vi "gyro_hand_display.vi"() -> ()   [LabVIEW 2019]
uses:
  SubVIs/Gyro_Reader/Controls/gyro_control_measurement_settings.ctl
panel:
  in  "Tab Control":enum32{"File IO", "Selection", "Time", "SNR"}(tab)
  in  "Missing GPX file":bool
  in  "Missing Hand file":bool
  in  "Missing Ship file":bool
  in  "GPX path":path
  in  "Hand path":path
  in  "Ship path":path
  in  "Old Akti File":bool
  out "hand data":waveform(dbl)[](graph)
  out "ship data":waveform(dbl)[](graph)
  in  "Sec":dbl=60.0
  in  "Start Cursor":timestamp
  in  "Reset Cursors":bool
  in  "GPS Offset":dbl
  out "GPS Graph":cluster{timestamp[], "Y":dbl[]}[](graph)
  in  "Read in Button":bool
  in  "Stop Button":bool
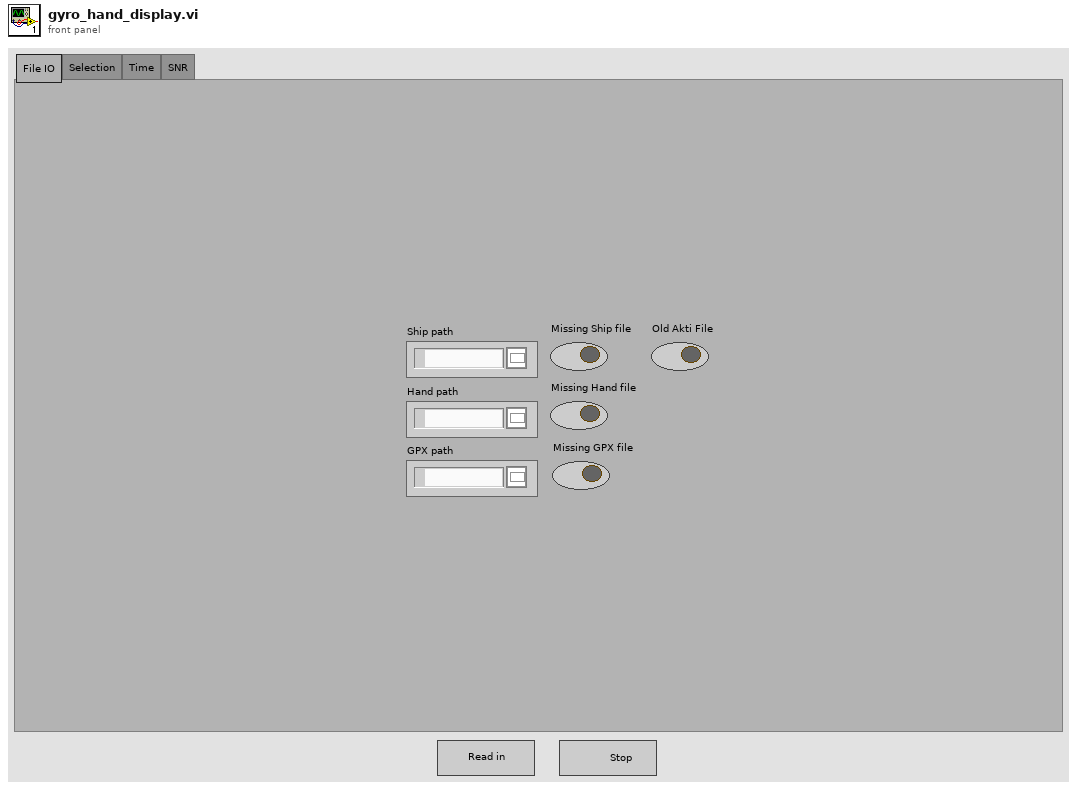
[diagram p1: front panel]
types:
  T1 = typedef "gyro_control_measurement_settings.ctl" = cluster{"# Pages":i32, "ODR":u8, "xlRange":u8, "gyroRange":u8, "id":u8, "Samplig Freq [Hz]":dbl, "xlRange in g":dbl, "gyroRange in dps":dbl}
  T2 = cluster{"IO Meta":cluster{"ship file missing?":bool, "hand file missing?":bool, "GPX file missing?":bool, "old akti file?":bool, "Start Time":timestamp, "GPS offset":dbl}, "Ship Data":cluster{"Ship Acceleration":waveform(dbl)[], "Ship Angular Velocity":waveform(dbl)[]}, "Hand Data":cluster{"Hand Acceleration":waveform(dbl)[], "Hand Angular Velocity":waveform(dbl)[]}, "Ship Meta":T1, "Hand Meta":T1, "GPS Data":cluster{"XY Speed data":cluster{"Array":timestamp[], "Array":dbl[]}, "Lat/Lon Position":cluster{"Array":timestamp[], "Array":dbl[], "Array":dbl[]}, "Position Graph":cluster{"X":dbl, "Y":dbl}[]}}
  T3 = typedef "LVRangeTypeDef.ctl" = cluster{"Minimum":dbl, "Maximum":dbl, "Increment":dbl, "Minor Increment":dbl, "Start":dbl}
  T4 = typedef "control_all_in_one_package.ctl" = cluster{"memory structure":T5, "actigraph settings":T6, "time informations":T7, "measurement data":T8}
  T5 = typedef "control_memory_structure.ctl" = cluster{"length of metadata [byte]":i32, "length of page [byte]":i32, "length of measurement data on page [byte]":i32, "length of dataset [byte]":i32}
  T6 = typedef "control_measurement_settings.ctl" = cluster{"sampling frequency [Hz]":dbl, "measurement interval [± g]":i32, "high precision?":bool, "number of pages":i32, "rate code":i32, "range code":i32, "id":i32}
  T7 = typedef "control_time_informations.ctl" = cluster{"starting time":timestamp, "ending time":timestamp, "dt[s]":dbl, "sampling rate [Hz]":dbl, "length":dbl}
  T8 = typedef "control_measurement_data.ctl" = cluster{"number of samples per axis":i32, "timestamp array":dbl[], "offset array":dbl[], "x, y, z axis data":waveform(dbl)[], "normalised magnitude of acceleartion vectors":waveform(dbl), "calibration coefficients":T9, "statistics":T10, "battery voltage":waveform(dbl), "magnitude of acceleartion vectors":waveform(dbl)}
  T9 = typedef "control_calibration_coefficients.ctl" = cluster{"Sx":dbl, "Ox":dbl, "Sy":dbl, "Oy":dbl, "Sz":dbl, "Oz":dbl}
  T10 = typedef "control_statistics.ctl" = cluster{"mean of x axis acceleration":dbl, "standard devation of x axis acceleration":dbl, "mean of y axis acceleration":dbl, "standard devation of y axis acceleration":dbl, "mean of z axis acceleration":dbl, "standard devation of z axis acceleration":dbl, "mean of normalised magnitude of acceleration":dbl, "standard devation of normalised magnitude of acceleration":dbl}
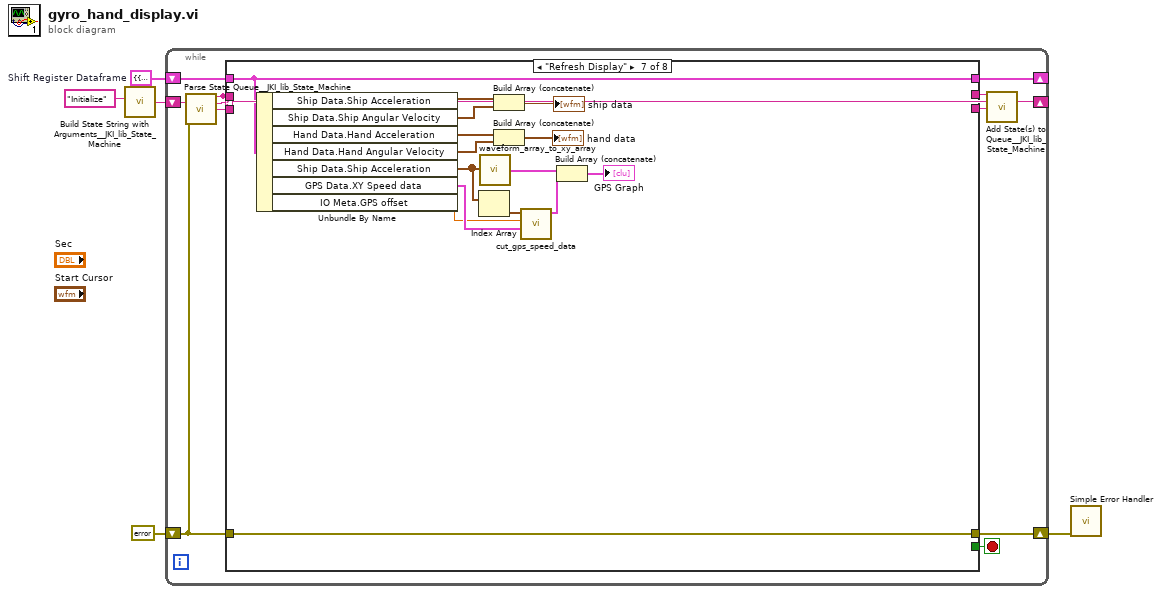
[diagram p0: block diagram]
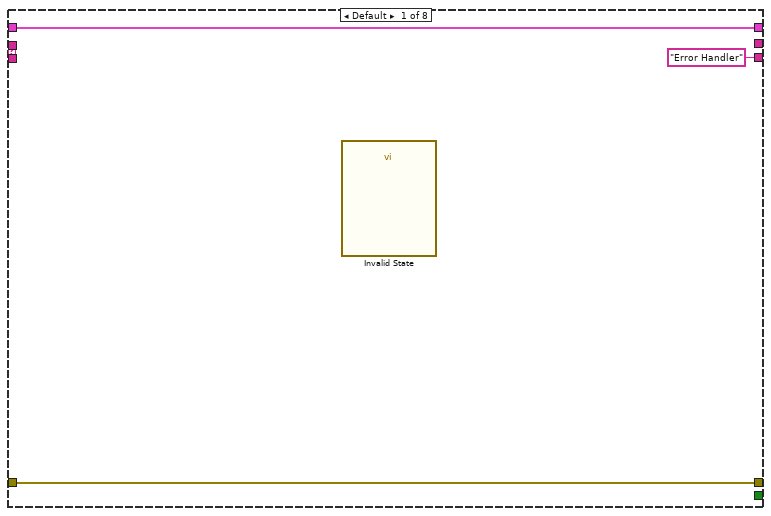
[diagram p2: hidden frame]
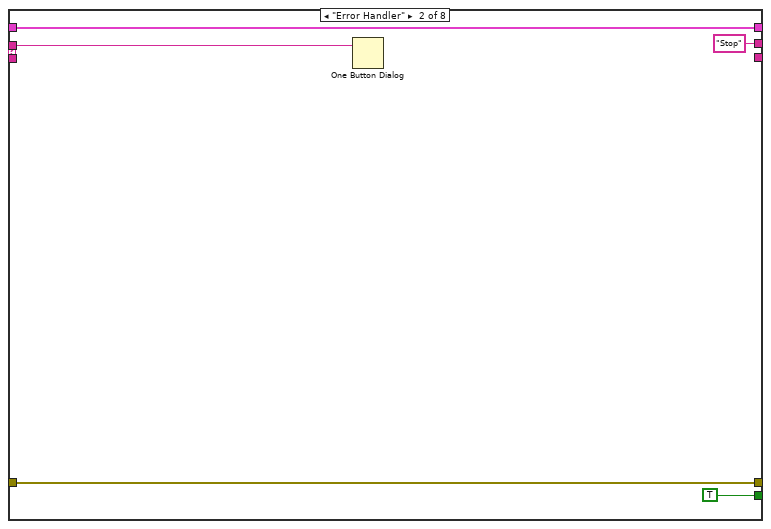
[diagram p3: hidden frame]
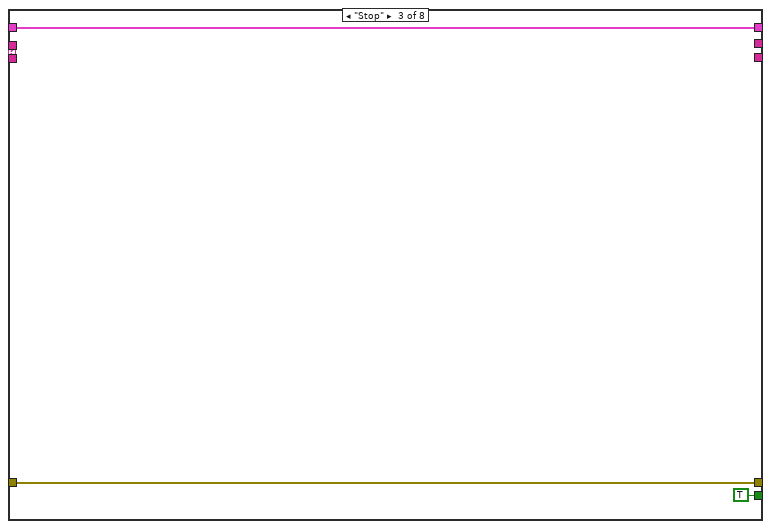
[diagram p4: hidden frame]
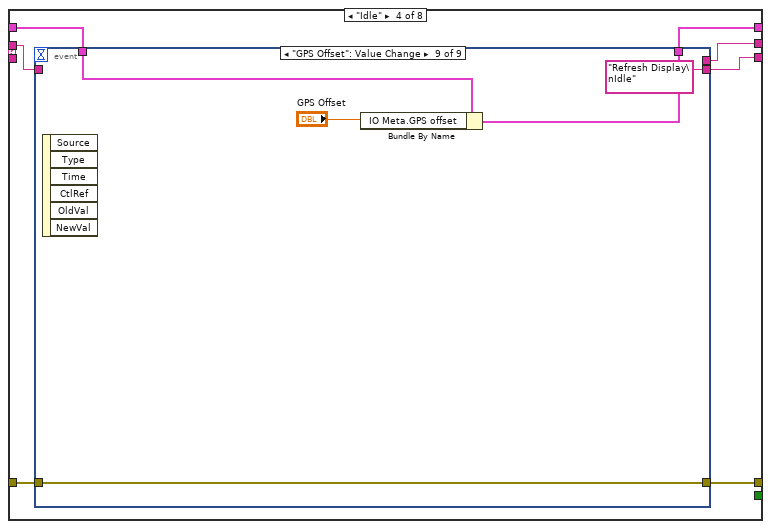
[diagram p5: hidden frame]
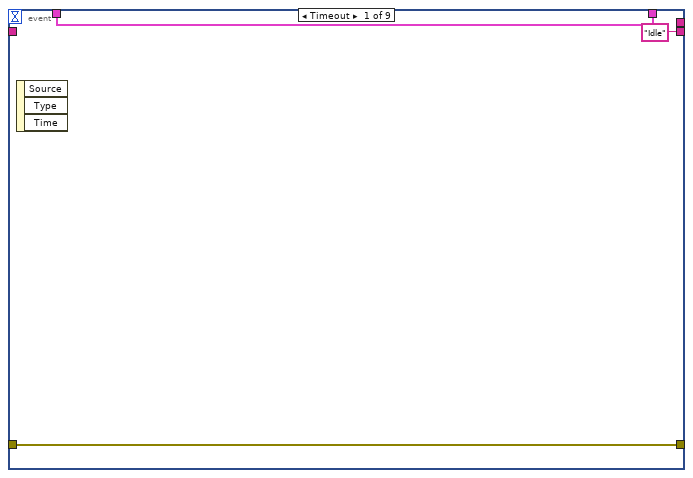
[diagram p6: hidden frame]
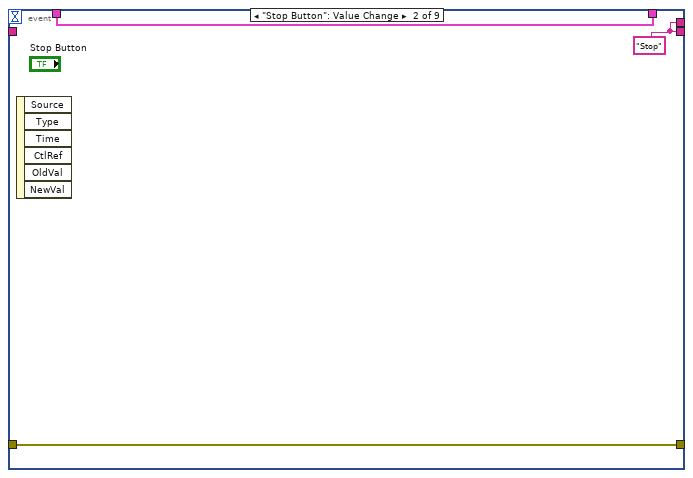
[diagram p7: hidden frame]
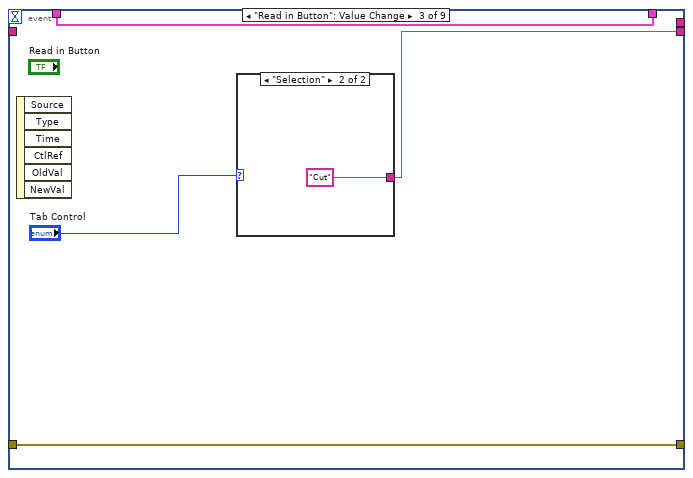
[diagram p8: hidden frame]
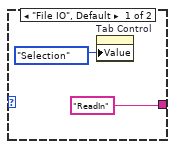
[diagram p9: hidden frame]
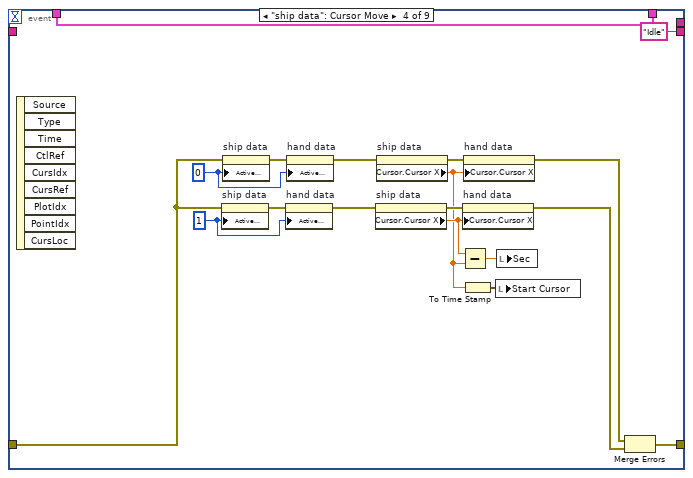
[diagram p10: hidden frame]
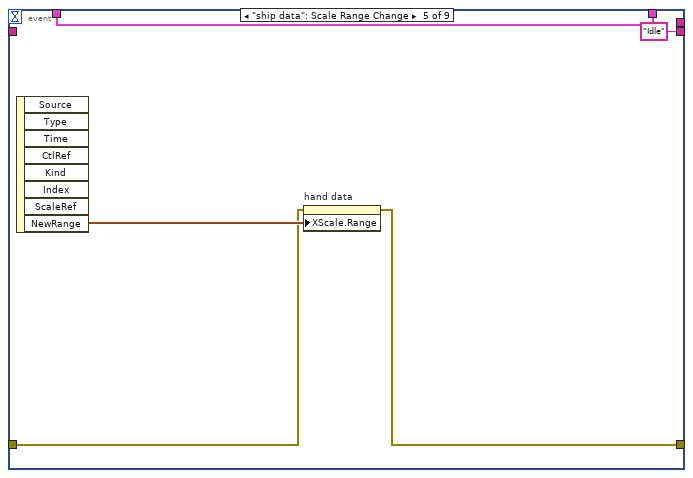
[diagram p11: hidden frame]
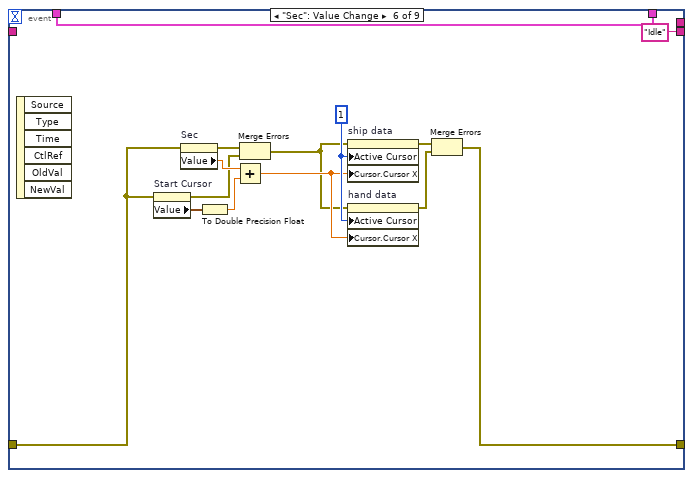
[diagram p12: hidden frame]
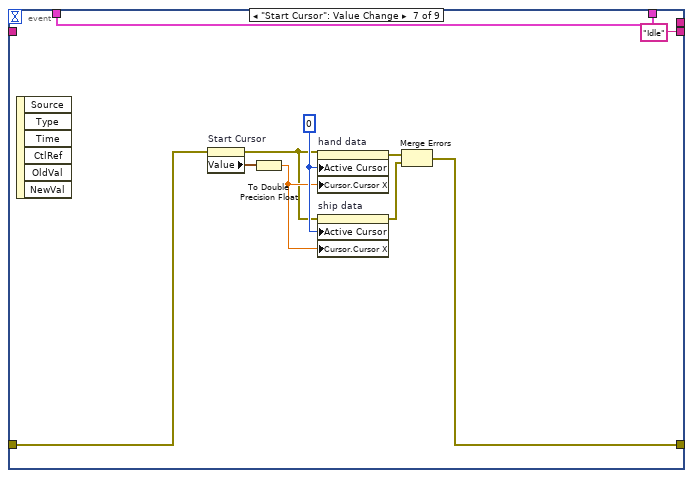
[diagram p13: hidden frame]
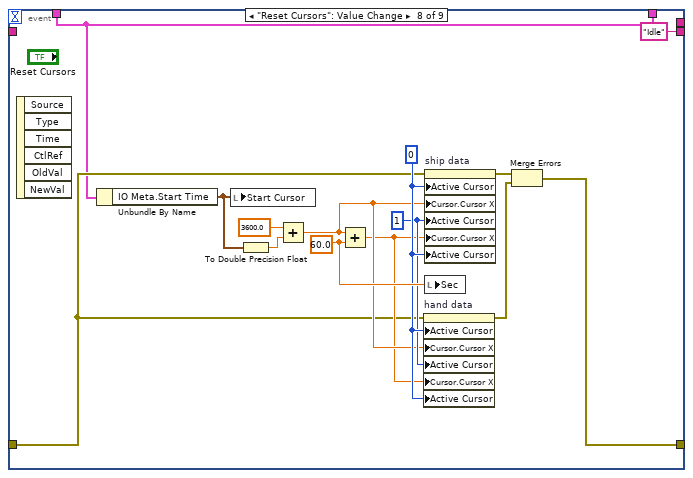
[diagram p14: hidden frame]
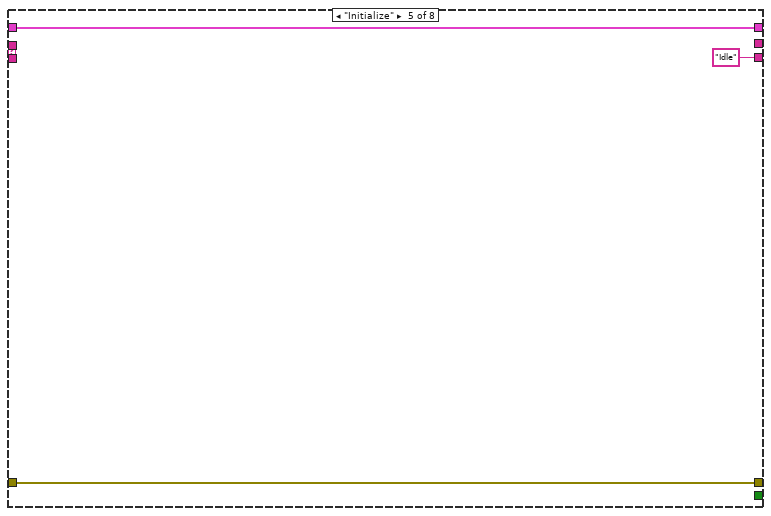
[diagram p15: hidden frame]
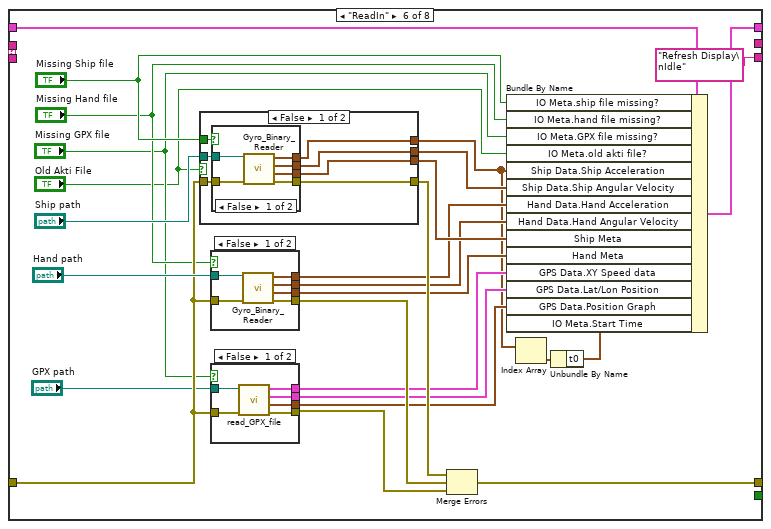
[diagram p16: hidden frame]
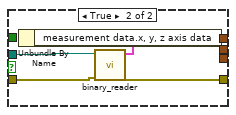
[diagram p20: hidden frame]
diagram:
  w1 = T2 {"IO Meta"={"ship file missing?"=TRUE, "hand file missing?"=TRUE, "GPX file missing?"=TRUE, "old akti file?"=FALSE, "Start Time"=timestamp(0 s since 1904-01-01), "GPS offset"=0.0}, "Ship Data"={"Ship Acceleration"=[], "Ship Angular Velocity"=[]}, "Hand Data"={"Hand Acceleration"=[], "Hand Angular Velocity"=[]}, "Ship Meta"={"# Pages"=0, "ODR"=0, "xlRange"=0, "gyroRange"=0, "id"=0, "Samplig Freq [Hz]"=9.980607627666451, "xlRange in g"=0.0, "gyroRange in dps"=0.0}, "Hand Meta"={"# Pages"=0, "ODR"=0, "xlRange"=0, "gyroRange"=0, "id"=0, "Samplig Freq [Hz]"=9.980607627666451, "xlRange in g"=0.0, "gyroRange in dps"=0.0}, "GPS Data"={"XY Speed data"={"Array"=[], "Array"=[]}, "Lat/Lon Position"={"Array"=[], "Array"=[], "Array"=[]}, "Position Graph"=[]}}  # Shift Register Dataframe
  n1 = call <vilib>:"Build State String with Arguments__JKI_lib_State_Machine.vi"("State"="Initialize") -> ("State with Arguments"=w5:string)  [unwired: 5 in]
  n2 = while {
    shift-right: [w14] -> w2
    shift-left: errorcluster {"status"=FALSE, "code"=0, "source"=""} ("error in (no error)") -> [w15]
    shift-right: [w7] -> _
    shift-left: w5 -> [w16]
    shift-right: [w9] -> _
    shift-left: w1 -> [w10]
    stop <- w17 stop-if-true
    n3 = call <vilib>:"Parse State Queue__JKI_lib_State_Machine.vi"("State Queue"=w16, "Error In (no error)"=w15) -> ("Remaining States"=w12:string, "Current State"=w13:string, "Arguments"=w11:string)  [unwired: 11 in]
    n4 = case shown="\"Refresh Display\"" w13 {
      tunnel: [_ TRUE TRUE _ _ _ _ _] -> w17
      tunnel: [w20 w24 w28 w35 w116 w141 w190 w192] -> w14
      tunnel: w15 -> [w20 w24 w28 w34 w116 w138 w190 w192]
      tunnel: w12 -> [_ w21 _ w33 _ _ _ _]
      tunnel: w11 -> [_ _ _ _ _ _ _ _]
      tunnel: w10 -> [w19 w23 w26 w30 w115 w117 w189 w193]
      tunnel: [w19 w23 w26 w29 w115 w134 w189 w193] -> w9
      tunnel: ["Error Handler" ("States Out") _ _ w32 "Idle" ("State(s) at Back (\"\")") "Refresh Display\nIdle" ("State(s) at Back (\"\")") _ "Idle" ("States Out")] -> w8
      tunnel: [_ "Stop" ("States Out") _ w31 _ _ _ _] -> w6
      frame Default {
        n5 = call "Invalid State"() -> ()  [unwired: 10 in, 2 out]
      }
      frame "Error Handler" {
        n6 = One Button Dialog(message=w21) -> ()  [unwired: 1 in, 1 out]
      }
      frame "Stop" {
      }
      frame "Idle" {
        n7 = event shown="[8] \"GPS Offset\": Value Change" {
          selector: _ -> [_ _ _ _ _ _ _ _ _]
          dyn-events: _ -> [_ _ _ _ _ _ _ _ _]
          timeout: _ -> [_ _ _ _ _ _ _ _ _]
          tunnel: w33 -> [_ _ _ _ _ _ _ _ _]
          tunnel: ["Idle" ("Remaining States") w40 w43 "Idle" ("Remaining States") "Idle" ("Remaining States") "Idle" ("Remaining States") "Idle" ("Remaining States") "Idle" ("Remaining States") "Refresh Display\nIdle" ("Remaining States")] -> w32
          tunnel: [w38 w41 w45 w58 w67 w78 w90 w96 w109] -> w35
          tunnel: w34 -> [w38 w41 w45 w60 w68 w72 w87 w99 w109]
          tunnel: [_ w40 _ _ _ _ _ _ _] -> w31
          tunnel: w30 -> [w36 w39 w42 w49 w66 w71 w85 w95 w113]
          tunnel: [w36 w39 w42 w49 w66 w71 w85 w95 w111] -> w29
          event Timeout {
            n8 = event-data() -> ()  [unwired: 1 in, 3 out]
          }
          event "Stop Button": Value Change {
            w40 = "Stop" ("Remaining States")
            n9 = event-data() -> ()  [unwired: 1 in, 6 out]
          }
          event "Read in Button": Value Change {
            n10 = event-data() -> ()  [unwired: 1 in, 6 out]
            n11 = case shown="\"Selection\"" "Tab Control" {
              tunnel: ["ReadIn" ("Remaining States") "Cut" ("Remaining States")] -> w43
              frame "File IO", Default {
                n12 = property on="Tab Control" class="TabCtl (strict)"("Value"=enum32{"File IO", "Selection", "Time", "SNR"}."Selection" ("Tab Control")) -> ()  [unwired: 2 in, 2 out]
              }
              frame "Selection" {
              }
            }
          }
          event "ship data": Cursor Move {
            w55 = 1
            w54 = 0
            n13 = event-data() -> ()  [unwired: 1 in, 9 out]
            n14 = property on="ship data" class="WFGraph (strict)"(error in=w60, "Active Cursor"=w55) -> (error out=w59:errorcluster)  [unwired: 1 in, 1 out]
            n15 = property on="ship data" class="WFGraph (strict)"("Active Cursor"=w54) -> ()  [unwired: 2 in, 2 out]
            n16 = property on="hand data" class="WFGraph (strict)"(error in=w59, "Active Cursor"=w55) -> (error out=w62:errorcluster)  [unwired: 1 in, 1 out]
            n17 = property on="hand data" class="WFGraph (strict)"(error in=w60, "Active Cursor"=w54) -> (error out=w64:errorcluster)  [unwired: 1 in, 1 out]
            n18 = property on="ship data" class="WFGraph (strict)"(error in=w62) -> (error out=w61:errorcluster, "Cursor.Cursor X"=w52:dbl)  [unwired: 1 in, 1 out]
            n19 = property on="ship data" class="WFGraph (strict)"(error in=w64) -> (error out=w65:errorcluster, "Cursor.Cursor X"=w50:dbl)  [unwired: 1 in, 1 out]
            n20 = Subtract(x=w52, y=w50) -> (x-y=w53:dbl)
            n21 = property on="hand data" class="WFGraph (strict)"(error in=w61, "Cursor.Cursor X"=w52) -> (error out=w56:errorcluster)  [unwired: 1 in, 1 out]
            n22 = To Time Stamp(1:w50) -> (0:w51:timestamp)
            n23 = property on="hand data" class="WFGraph (strict)"(error in=w65, "Cursor.Cursor X"=w50) -> (error out=w57:errorcluster)  [unwired: 1 in, 1 out]
            n24 = local write "Start Cursor"(w51) -> ()
            n25 = local write "Sec"(w53) -> ()
            n26 = Merge Errors(w57, w56) -> (w58:errorcluster)
          }
          event "ship data": Scale Range Change {
            n27 = event-data() -> ("NewRange"=w70:T3)  [unwired: 1 in, 7 out]
            n28 = property on="hand data" class="WFGraph (strict)"(error in=w68, "XScale.Range"=w70) -> (error out=w67:errorcluster)  [unwired: 1 in, 1 out]
          }
          event "Sec": Value Change {
            w82 = u32 1 ("Active Cursor")
            n29 = event-data() -> ()  [unwired: 1 in, 6 out]
            n30 = property on="Start Cursor" class="AbsTime (strict)"(error in=w72) -> (error out=w73:errorcluster, "Value"=w74:timestamp)  [unwired: 1 in, 1 out]
            n31 = property on="Sec" class="DigNum (strict)"(error in=w72) -> (error out=w77:errorcluster, "Value"=w83:dbl)  [unwired: 1 in, 1 out]
            n32 = To Double Precision Float(number=w74) -> (double precision float=w84:dbl)
            n33 = Add(x=w83, y=w84) -> (x+y=w81:dbl)
            n34 = Merge Errors(w77, w73) -> (w76:errorcluster)
            n35 = property on="ship data" class="WFGraph (strict)"(error in=w76, "Active Cursor"=w82, "Cursor.Cursor X"=w81) -> (error out=w80:errorcluster)  [unwired: 1 in, 1 out]
            n36 = property on="hand data" class="WFGraph (strict)"(error in=w76, "Active Cursor"=w82, "Cursor.Cursor X"=w81) -> (error out=w79:errorcluster)  [unwired: 1 in, 1 out]
            n37 = Merge Errors(w80, w79) -> (w78:errorcluster)
          }
          event "Start Cursor": Value Change {
            w92 = u32 0 ("Active Cursor")
            n38 = event-data() -> ()  [unwired: 1 in, 6 out]
            n39 = property on="Start Cursor" class="AbsTime (strict)"(error in=w87) -> (error out=w88:errorcluster, "Value"=w86:timestamp)  [unwired: 1 in, 1 out]
            n40 = To Double Precision Float(number=w86) -> (double precision float=w91:dbl)
            n41 = property on="hand data" class="WFGraph (strict)"(error in=w88, "Active Cursor"=w92, "Cursor.Cursor X"=w91) -> (error out=w93:errorcluster)  [unwired: 1 in, 1 out]
            n42 = property on="ship data" class="WFGraph (strict)"(error in=w88, "Active Cursor"=w92, "Cursor.Cursor X"=w91) -> (error out=w94:errorcluster)  [unwired: 1 in, 1 out]
            n43 = Merge Errors(w93, w94) -> (w90:errorcluster)
          }
          event "Reset Cursors": Value Change {
            w105 = 60.0 ("y")
            w103 = 1
            w104 = 0
            n44 = event-data() -> ()  [unwired: 1 in, 6 out]
            n45 = Unbundle By Name(w95) -> ("IO Meta.Start Time"=w100:timestamp)
            n46 = local write "Start Cursor"(w100) -> ()
            n47 = To Double Precision Float(number=w100) -> (double precision float=w106:dbl)
            n48 = Add(x=3600.0, y=w106) -> (x+y=w102:dbl)
            n49 = Add(x=w102, y=w105) -> (x+y=w101:dbl)
            n50 = property on="hand data" class="WFGraph (strict)"(error in=w99, "Active Cursor"=w104, "Cursor.Cursor X"=w102, "Active Cursor"=w103, "Cursor.Cursor X"=w101, "Active Cursor"=w104) -> (error out=w97:errorcluster)  [unwired: 1 in, 1 out]
            n51 = property on="ship data" class="WFGraph (strict)"(error in=w99, "Active Cursor"=w104, "Cursor.Cursor X"=w102, "Active Cursor"=w103, "Cursor.Cursor X"=w101, "Active Cursor"=w104) -> (error out=w98:errorcluster)  [unwired: 1 in, 1 out]
            n52 = local write "Sec"(w105) -> ()
            n53 = Merge Errors(w98, w97) -> (w96:errorcluster)
          }
          event "GPS Offset": Value Change {
            n54 = event-data() -> ()  [unwired: 1 in, 6 out]
            n55 = Bundle By Name(cluster=w113, "IO Meta.GPS offset"="GPS Offset") -> (w111:T2)
          }
        }
      }
      frame "Initialize" {
      }
      frame "ReadIn" {
        n56 = case shown="False" "Old Akti File" {
          tunnel: "Missing Ship file" -> [w163 _]
          tunnel: "Ship path" -> [w162 w174]
          tunnel: w138 -> [w161 w172]
          tunnel: [w160 w173] -> w140
          tunnel: [w159 w171] -> w120
          tunnel: [w158 _] -> w128
          tunnel: [w157 _] -> w127
          frame False {
            n57 = case shown="False" w163 {
              tunnel: w162 -> [w169 _]
              tunnel: w161 -> [w168 w170]
              tunnel: [w167 w170] -> w160
              tunnel: [w166 _] -> w159
              tunnel: [w165 _] -> w158
              tunnel: [w164 _] -> w157
              frame False {
                n58 = call "Gyro_Binary_Reader.vi"("error in"=w168, "file path (use dialog)"=w169) -> ("error out"=w167:errorcluster, "Meta"=w164:T1, "Angular Velocity"=w165:waveform(dbl)[], "Acceleration"=w166:waveform(dbl)[])  [unwired: 6 in]
              }
              frame True {
              }
            }
          }
          frame True {
            n59 = call "binary_reader.vi"("error in"=w172, "path to binary file"=w174) -> ("error out"=w173:errorcluster, "all in one package"=w175:T4)  [unwired: 6 in, 1 out]
            n60 = Unbundle By Name(w175) -> ("measurement data.x, y, z axis data"=w171:waveform(dbl)[])
          }
        }
        n61 = case shown="False" "Missing Hand file" {
          tunnel: "Hand path" -> [w155 _]
          tunnel: w138 -> [w154 w156]
          tunnel: [w153 w156] -> w136
          tunnel: [w152 _] -> w126
          tunnel: [w151 _] -> w125
          tunnel: [w150 _] -> w124
          frame False {
            n62 = call "Gyro_Binary_Reader.vi"("error in"=w154, "file path (use dialog)"=w155) -> ("error out"=w153:errorcluster, "Meta"=w150:T1, "Angular Velocity"=w151:waveform(dbl)[], "Acceleration"=w152:waveform(dbl)[])  [unwired: 6 in]
          }
          frame True {
          }
        }
        n63 = case shown="False" "Missing GPX file" {
          tunnel: "GPX path" -> [w148 _]
          tunnel: w138 -> [w147 w149]
          tunnel: [w146 w149] -> w135
          tunnel: [w145 _] -> w123
          tunnel: [w144 _] -> w122
          tunnel: [w143 _] -> w121
          frame False {
            n64 = call "read_GPX_file.vi"("error in"=w147, "GPX File Path"=w148) -> ("error out"=w146:errorcluster, "position Graph"=w143:cluster{"X":dbl, "Y":dbl}[], "lat/lon position"=w144:cluster{timestamp[], dbl[], dbl[]}, "XY Speed data"=w145:cluster{timestamp[], dbl[]})  [unwired: 2 in]
          }
          frame True {
          }
        }
        n65 = Merge Errors(w140, w136, w135) -> (w141:errorcluster)
        n66 = Index Array(array=w120) -> (element=w119:waveform(dbl))  [unwired: 1 in]
        n67 = Unbundle By Name(w119) -> ("t0"=w118:timestamp)
        n68 = Bundle By Name(cluster=w117, "IO Meta.ship file missing?"="Missing Ship file", "IO Meta.hand file missing?"="Missing Hand file", "IO Meta.GPX file missing?"="Missing GPX file", "IO Meta.old akti file?"="Old Akti File", "Ship Data.Ship Acceleration"=w120, "Ship Data.Ship Angular Velocity"=w128, "Hand Data.Hand Acceleration"=w126, "Hand Data.Hand Angular Velocity"=w125, "Ship Meta"=w127, "Hand Meta"=w124, "GPS Data.XY Speed data"=w123, "GPS Data.Lat/Lon Position"=w122, "GPS Data.Position Graph"=w121, "IO Meta.Start Time"=w118) -> (w134:T2)
      }
      frame "Refresh Display" {
        n69 = Unbundle By Name(w189) -> ("Ship Data.Ship Acceleration"=w188:waveform(dbl)[], "Ship Data.Ship Angular Velocity"=w187:waveform(dbl)[], "Hand Data.Hand Acceleration"=w185:waveform(dbl)[], "Hand Data.Hand Angular Velocity"=w184:waveform(dbl)[], "Ship Data.Ship Acceleration"=w179:waveform(dbl)[], "GPS Data.XY Speed data"=w181:cluster{"Array":timestamp[], "Array":dbl[]}, "IO Meta.GPS offset"=w180:dbl)
        n70 = Index Array(array=w179) -> (element=w178:waveform(dbl))  [unwired: 1 in]
        n71 = call "waveform_array_to_xy_array.vi"("waveform array"=w179) -> ("XY array"=w177:cluster{timestamp[], "Y":dbl[]}[])
        n72 = Build Array (concatenate)(w188, w187) -> (→"ship data":waveform(dbl)[])
        n73 = Build Array (concatenate)(w185, w184) -> (→"hand data":waveform(dbl)[])
        n74 = call "cut_gps_speed_data.vi"("timestamp gps speed data"=w181, "gps shift [s]"=w180, "acc data"=w178) -> ("XY gps speed data"=w176:cluster{dbl[], dbl[]})  [unwired: 8 in]
        n75 = Build Array (concatenate)(w177, w176) -> (→"GPS Graph":cluster{timestamp[], "Y":dbl[]}[])
      }
      frame "Cut" {
        n76 = call "Display Message to User"() -> ()  [unwired: 10 in, 2 out]
      }
    }
    n77 = call <vilib>:"Add State(s) to Queue__JKI_lib_State_Machine.vi"("State(s) in Front (\"\")"=w6, "State(s) in (\"\")"=w12, "State(s) at Back (\"\")"=w8) -> ("States Out"=w7:string)  [unwired: 12 in]
  }
  n78 = call <vilib>:"Simple Error Handler.vi"("error in (no error)"=w2) -> ()  [unwired: 4 in, 5 out]
